vi "acquisition.vi"(1 "samples per acquisition":dbl, 3 "sampling rate":dbl) -> ()   [LabVIEW 2014]
panel:
  out "Waveform Graph origin":dbl[](graph)
  in  "OK Button":bool
  out "Waveform Graph":dbl[](graph)
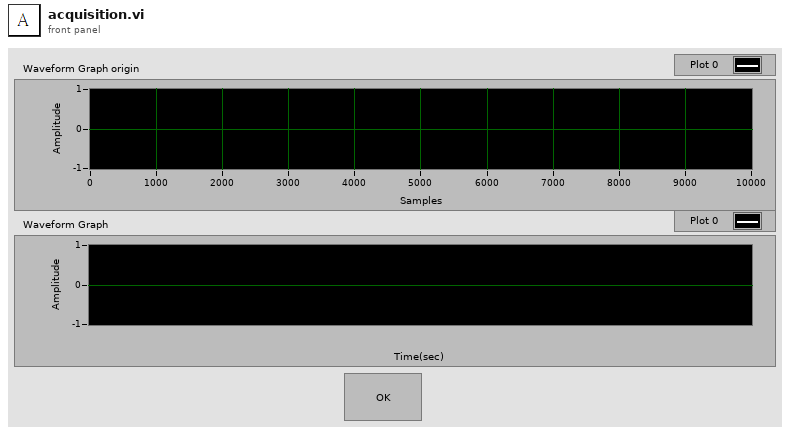
[diagram p1: front panel]
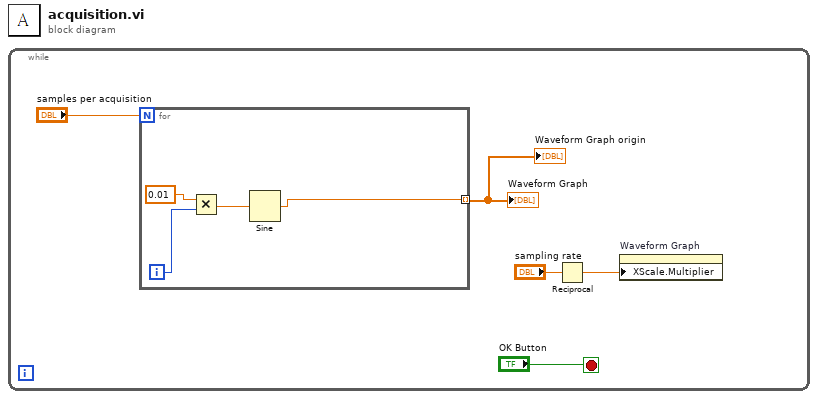
[diagram p0: block diagram]
diagram:
  n1 = while {
    stop <- "OK Button" stop-if-true
    n2 = for {
      N: "samples per acquisition" -> [_]
      tunnel: [w6] -> w1 mode=indexing
      i -> [w9]
      n3 = Multiply(x=0.01, y=w9) -> (x*y=w8:dbl)
      n4 = Sine(x=w8) -> (sin(x)=w6:dbl)
    }
    "Waveform Graph" <- w1
    "Waveform Graph origin" <- w1
    n5 = Reciprocal(x="sampling rate") -> (1/x=w3:dbl)
    n6 = property on="Waveform Graph" class="WFGraph (strict)"("XScale.Multiplier"=w3) -> ()  [unwired: 2 in, 2 out]
  }
